vi "ServoControl_myrio_v2.vi"() -> ()   [LabVIEW 2019]
uses:
  <vilib>/Utility/file.llb/Write Delimited Spreadsheet (DBL).vi
  <vilib>/Waveform/WDTFileIO.llb/Export Waveforms To Spreadsheet File (1D).vi
panel:
  in  "Frequency":dbl=0.1
  out "Numeric":dbl
  out "Sine":dynamicdata(graph)
  in  "Period":i64
  out "iteration":i32
  out "time":dbl
  in  "const/sine":bool
  in  "const  position":dbl=180.0
  out "sine position":dbl
  in  "file path (dialog if empty)":path
  in  "format (%.3f)":string="%.3f"
  out "position":cluster{dbl, dbl}(graph)
  out "resulting string":string
  in  "stop":bool
  out "read buffer":string
  out "error out 2":errorcluster
  in  "Baud rate 2":dbl=500000.0
  in  "VISA resource name 2":refnum<visa-resource-name>="ASRL1::INSTR"
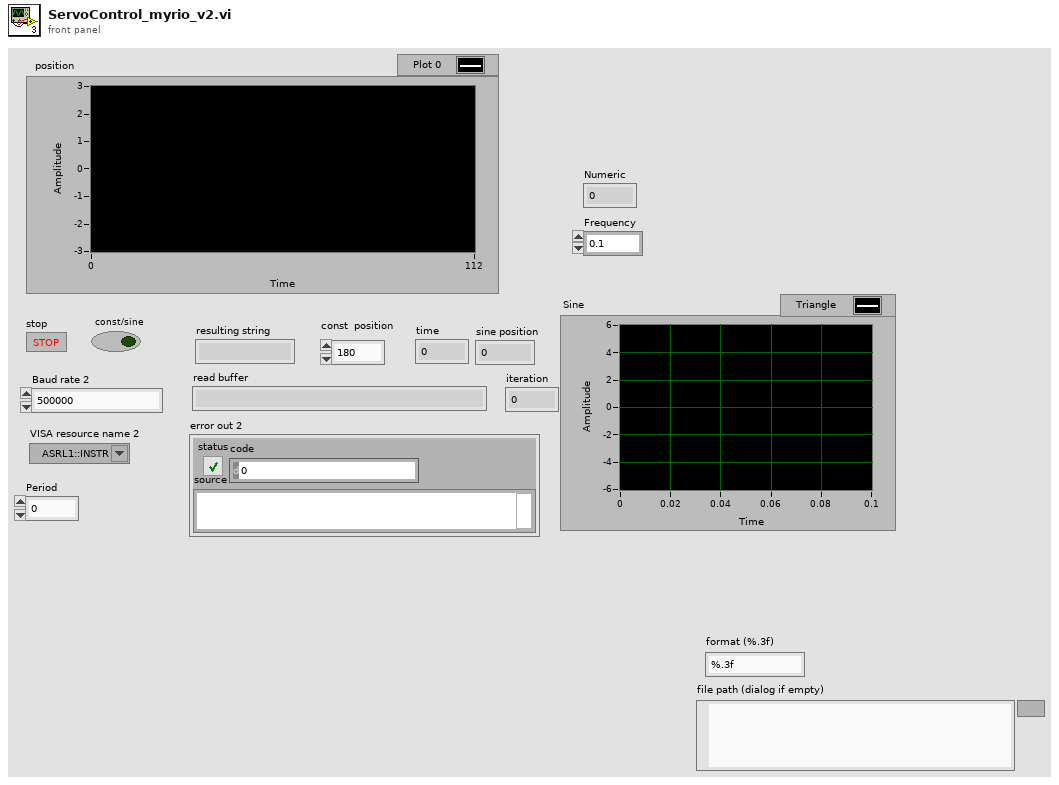
[diagram p1: front panel]
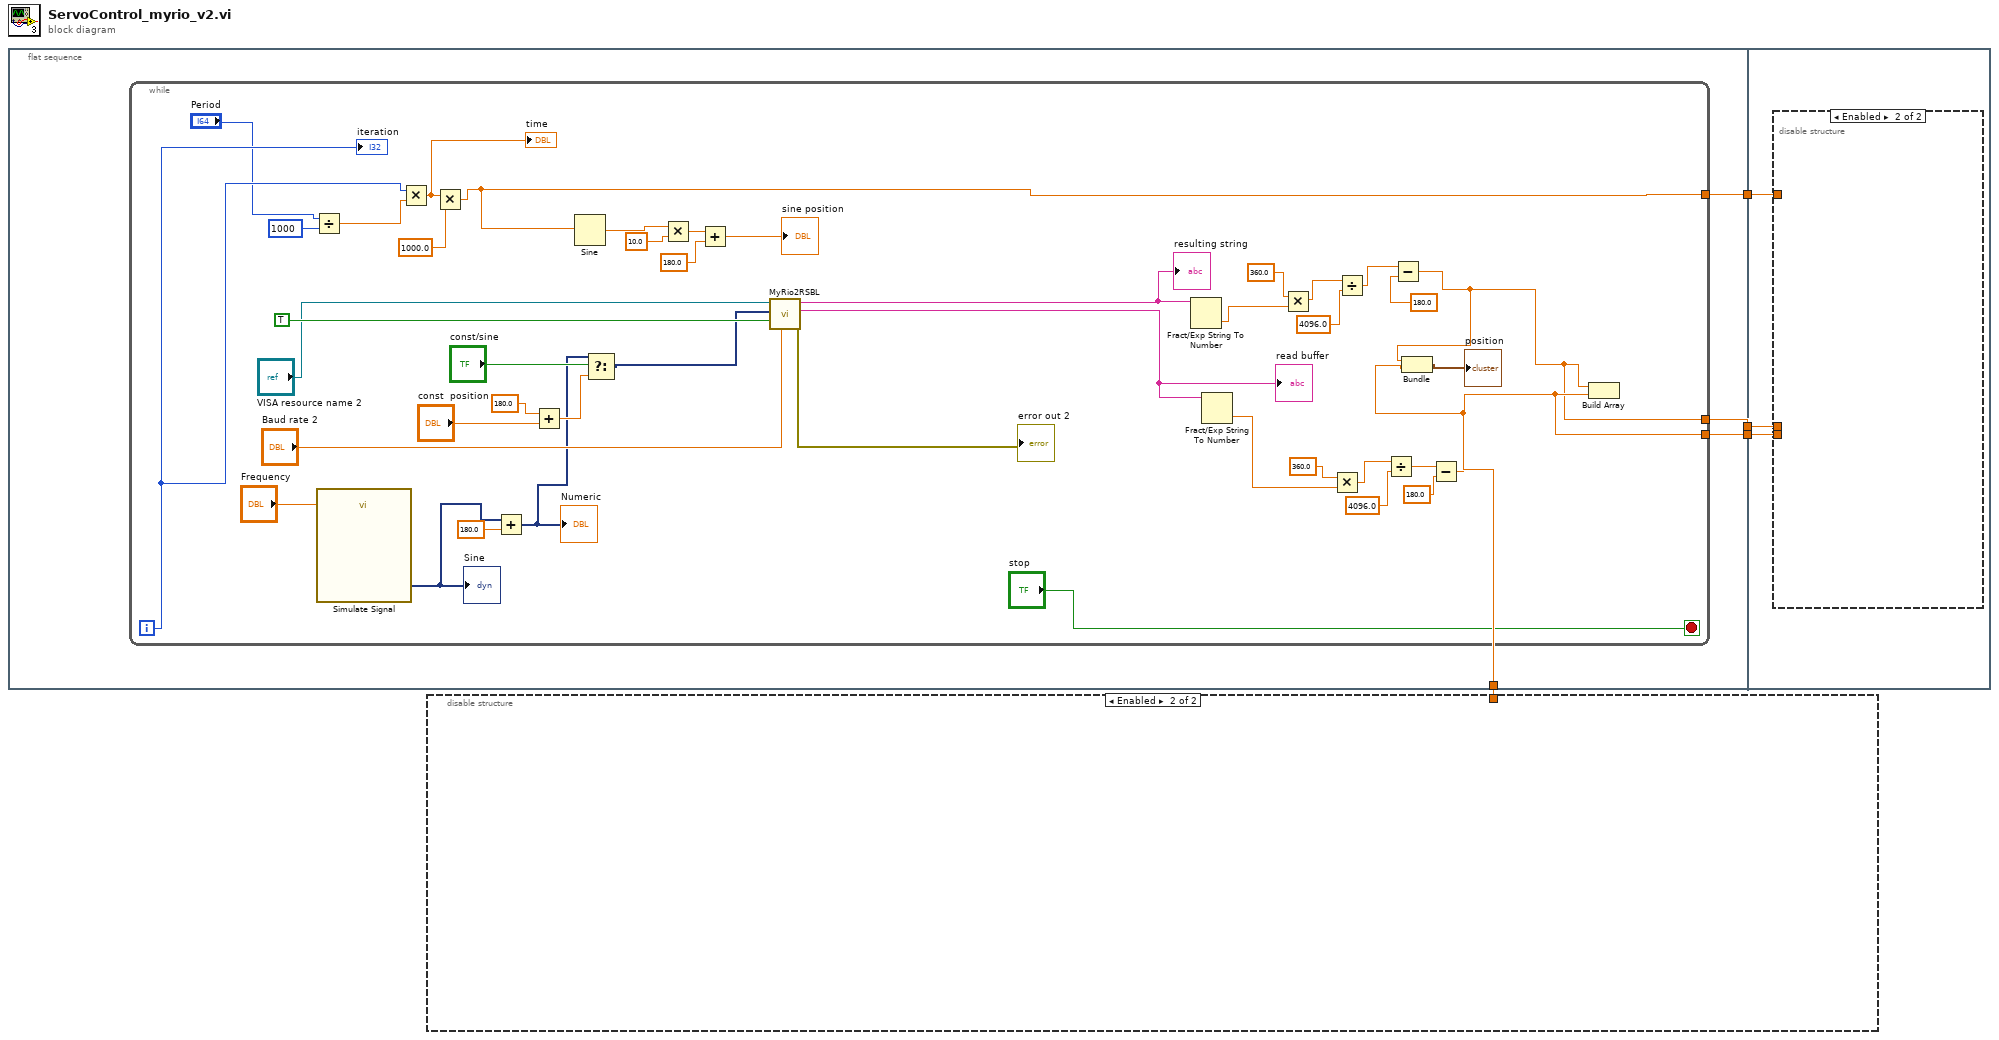
[diagram p0: block diagram]
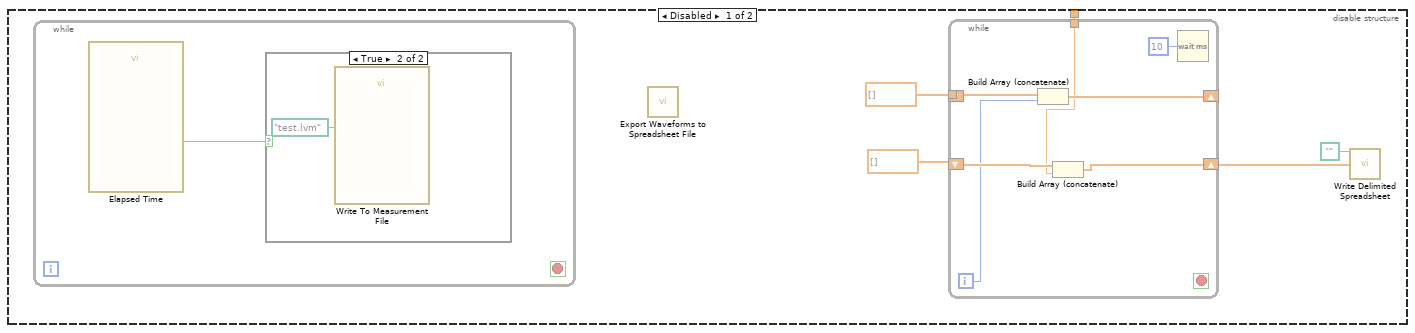
[diagram p2: hidden frame]
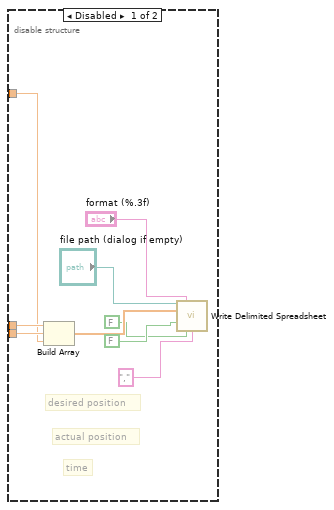
[diagram p4: hidden frame]
diagram:
  n1 = flat-sequence {
    tunnel: [w7] -> w4
    tunnel: [w5] -> w3
    tunnel: [w6] -> w2
    tunnel: [w5] -> w1
    tunnel: w4 -> [w53]
    tunnel: w3 -> [w52]
    tunnel: w2 -> [w51]
    frame #0 {
      n2 = while {
        tunnel: [w8] -> w7
        tunnel: [w50] -> w6
        tunnel: [w49] -> w5
        i -> [w15]
        stop <- "stop" stop-if-true
        n3 = Divide(x="Period", y=i64 1000) -> (x/y=w20:dbl)
        n4 = call "Simulate Signal"("Frequency"="Frequency") -> ("Triangle"=w11:dynamicdata)  [unwired: 13 in, 1 out]
        "Sine" <- w11
        n5 = Multiply(x=w15, y=w20) -> (x*y=w17:dbl)
        "time" <- w17
        n6 = Multiply(x=w17, y=1000.0) -> (x*y=w50:dbl)
        n7 = Add(x=w11, y=180.0) -> (x+y=w10:dynamicdata)
        "Numeric" <- w10
        n8 = Add(x=180.0, y="const  position") -> (x+y=w22:dbl)
        n9 = Sine(x=w50) -> (sin(x)=w42:dbl)
        n10 = Select(t=w10, s="const/sine", f=w22) -> (s? t:f=w38:dynamicdata)
        n11 = Multiply(x=w42, y=10.0) -> (x*y=w40:dbl)
        n12 = Add(x=w40, y=180.0) -> (x+y=→"sine position":dbl)
        n13 = call "MyRio2RSBL.vi"("Baud rate in"="Baud rate 2", "Boolean"=TRUE, "Numeric"=w38, "VISA Refnum in"="VISA resource name 2") -> ("error out"=→"error out 2":errorcluster, "read buffer"=w44:string, "String"=w43:string)  [unwired: 5 in]
        "resulting string" <- w43
        "read buffer" <- w44
        n14 = Fract/Exp String To Number(string=w43) -> (number=w30:dbl)  [unwired: 3 in, 1 out]
        n15 = Fract/Exp String To Number(string=w44) -> (number=w27:dbl)  [unwired: 3 in, 1 out]
        n16 = Multiply(x=360.0, y=w30) -> (x*y=w35:dbl)
        n17 = Multiply(x=360.0, y=w27) -> (x*y=w31:dbl)
        n18 = Divide(x=w35, y=4096.0) -> (x/y=w28:dbl)
        n19 = Divide(x=w31, y=4096.0) -> (x/y=w25:dbl)
        n20 = Subtract(x=w28, y=180.0) -> (x-y=w8:dbl)
        n21 = Subtract(x=w25, y=180.0) -> (x-y=w49:dbl)
        n22 = Bundle(w8, w49) -> (→"position":cluster{dbl, dbl})  [unwired: 1 in]
        n23 = Build Array(w8, w49) -> ()  [unwired: 1 out]
        "iteration" <- w15
      }
    }
    frame #1 {
      n24 = disable-structure shown="Enabled" {
        disable-tunnel: w53 -> [w62 _]
        disable-tunnel: w52 -> [w61 _]
        disable-tunnel: w51 -> [w60 _]
        frame Disabled {
          # "time"
          # "actual position"
          # "desired position"
          n25 = Build Array(w62, w61, w60) -> (w57:dbl[])
          n26 = call-poly <vilib>:"Write Delimited Spreadsheet.vi"("file path (dialog if empty)"="file path (dialog if empty)", "format (%.3f)"="format (%.3f)", "2D data"=w57, "append to file? (new file:F)"=FALSE ("transpose? (no:F)"), "transpose? (no:F)"=FALSE ("append to file? (new file:F)"), "delimiter (\\t)"="," ("delimiter (\\t)")) -> ()  [unwired: 8 in, 2 out]
        }
        frame Enabled {
        }
      }
    }
  }
  n27 = disable-structure shown="Enabled" {
    disable-tunnel: w1 -> [w65 _]
    frame Disabled {
      n28 = while {
        stop <- _ stop-if-true
        n29 = call "Elapsed Time"() -> ("Time has Elapsed"=w75:bool)  [unwired: 12 in, 7 out]
        n30 = case shown="True" w75 {
          frame False {
          }
          frame True {
            n31 = call "Write To Measurement File"("Filename"=path "test.lvm") -> ()  [unwired: 16 in, 3 out]
          }
        }
      }
      n32 = call-poly <vilib>:"Export Waveforms to Spreadsheet File.vi"() -> ()  [unwired: 10 in, 2 out]
      n33 = while {
        tunnel: dbl[] [] ("element") -> [w74]
        shift-right: [w73] -> _
        shift-left: _ -> [_]
        shift-right: [w70] -> w64
        shift-left: dbl[] [] ("element") -> [w71]
        tunnel: w65 -> [w68]
        i -> [w69]
        stop <- _ stop-if-true
        n34 = Build Array (concatenate)(w74, w69) -> (w73:dbl[])
        n35 = Build Array (concatenate)(w71, w68) -> (w70:dbl[])
        n36 = Wait (ms)(milliseconds to wait=u32 10) -> ()  [unwired: 1 out]
      }
      n37 = call-poly <vilib>:"Write Delimited Spreadsheet.vi"("file path (dialog if empty)"=path "", "1D data"=w64) -> ()  [unwired: 12 in, 2 out]
    }
    frame Enabled {
    }
  }
